vi "Increment Filename changename.vi"(8 "error in (no error)":errorcluster, 11 "path":path=path "C:/user/patrick/test/test/filename.itx") -> (0 "error out":errorcluster, 3 "modified path":path=path "C:/")   [LabVIEW 2016]
panel:
  out "Numeric":i32
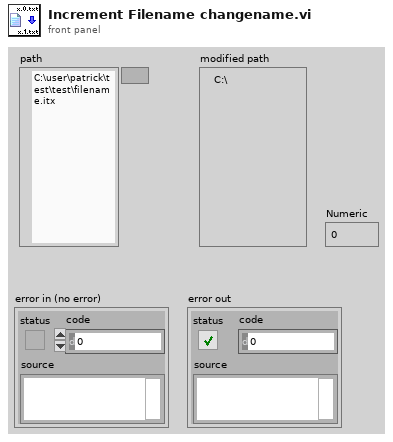
[diagram p1: front panel]
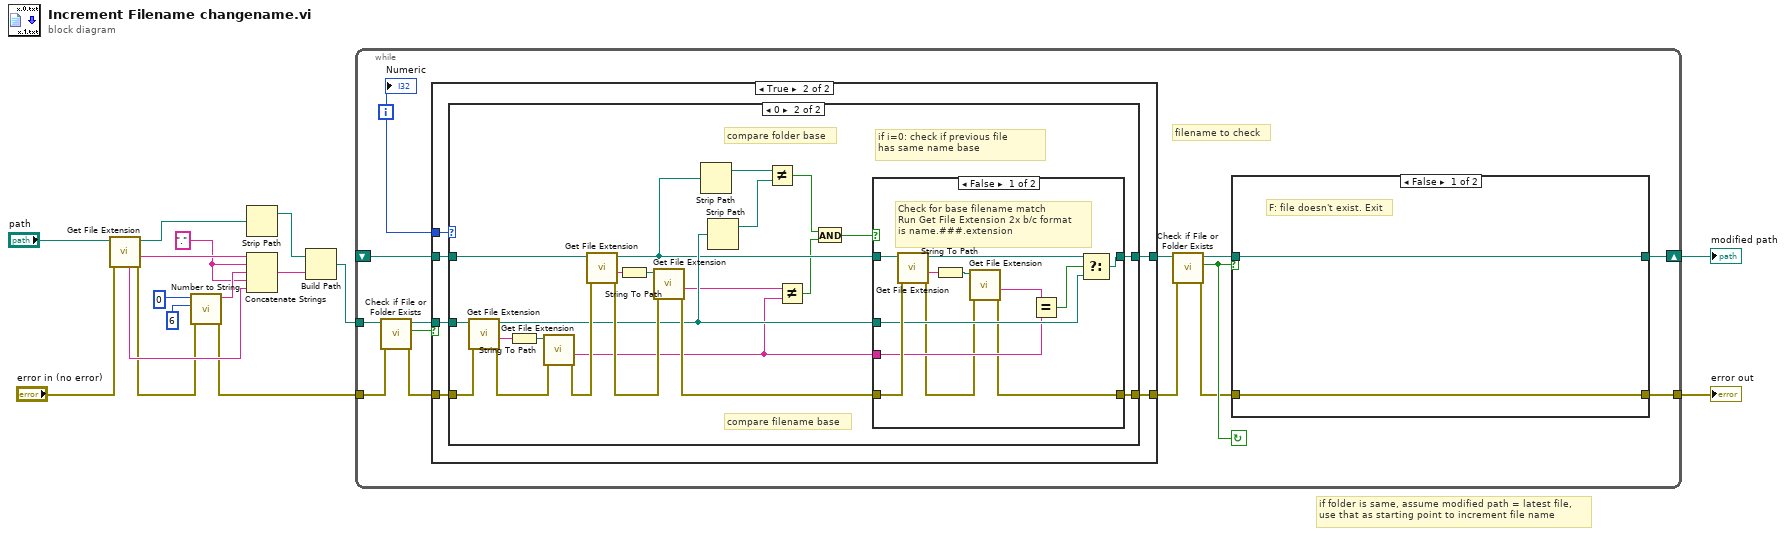
[diagram p0: block diagram]
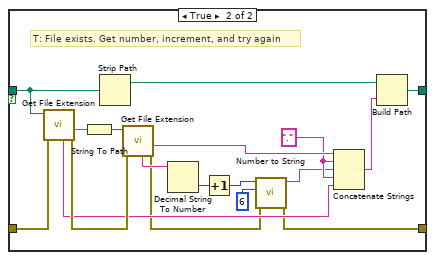
[diagram p5: hidden frame]
diagram:
  w4 = "."
  # "if folder is same, assume modified path = latest file,\nuse that as starting point to increment file name"
  n1 = call <vilib>:"Get File Extension.vi"("error in (no error)"="error in (no error)", "file"="path") -> ("error out"=w3:errorcluster, "filename without extension"=w11:string, "dup file"=w15:path, "unmodified file extension"=w8:string)  [unwired: 6 out]
  n2 = call "Number to String.vi"("error in (no error)"=w3, "desired minimum string length"=6, "number"=0) -> ("error out"=w2:errorcluster, "String"=w5:string)  [unwired: 7 in]
  n3 = Strip Path(path=w15) -> (stripped path=w7:path)  [unwired: 1 out]
  n4 = Concatenate Strings(w11, w4, w5, w4, w8) -> (w14:string)
  n5 = Build Path(base path=w7, name or relative path=w14) -> (appended path=w9:path)
  n6 = while {
    shift-right: [w28] -> w13
    shift-left: _ -> [w23]
    tunnel: w2 -> [w19]
    tunnel: [w26] -> w10
    tunnel: w9 -> [w20]
    i -> [w22]
    stop <- w29 continue-if-true
    # "filename to check"
    n7 = call <vilib>:"Check if File or Folder Exists.vi"("error in (no error)"=w19, "path"=w20) -> ("error out"=w18:errorcluster, "file or folder exists?"=w17:bool, "dup path"=w21:path)  [unwired: 7 out]
    n8 = case shown="True" w17 {
      tunnel: [w32 w38] -> w25
      tunnel: [w31 w37] -> w24
      tunnel: w23 -> [_ w36]
      tunnel: w22 -> [_ w35]
      tunnel: w21 -> [w31 w34]
      tunnel: w18 -> [w32 w33]
      frame False {
        # "If file.000000.* doesn't exist, just skip this step"
      }
      frame True {
        n9 = case shown="0" w35 {
          tunnel: [w39 w62] -> w38
          tunnel: w34 -> [_ w56]
          tunnel: w33 -> [w39 w61]
          tunnel: [w40 w60] -> w37
          tunnel: w36 -> [w40 w53]
          frame Default {
            # "if i>0, you can't use previous file and you're going to have to scan through\nthe entire directory"
          }
          frame 0 {
            # "compare filename base"
            # "compare folder base"
            # "if i=0: check if previous file\nhas same name base"
            n10 = call <vilib>:"Get File Extension.vi"("error in (no error)"=w61, "file"=w56) -> ("error out"=w57:errorcluster, "filename without extension"=w58:string, "dup file"=w47:path)  [unwired: 7 out]
            n11 = String To Path(string=w58) -> (path=w59:path)
            n12 = call <vilib>:"Get File Extension.vi"("error in (no error)"=w57, "file"=w59) -> ("error out"=w50:errorcluster, "filename without extension"=w44:string)  [unwired: 8 out]
            n13 = call <vilib>:"Get File Extension.vi"("error in (no error)"=w50, "file"=w53) -> ("error out"=w48:errorcluster, "filename without extension"=w52:string, "dup file"=w46:path)  [unwired: 7 out]
            n14 = String To Path(string=w52) -> (path=w51:path)
            n15 = call <vilib>:"Get File Extension.vi"("error in (no error)"=w48, "file"=w51) -> ("error out"=w49:errorcluster, "filename without extension"=w45:string)  [unwired: 8 out]
            n16 = Strip Path(path=w46) -> (stripped path=w54:path)  [unwired: 1 out]
            n17 = Strip Path(path=w47) -> (stripped path=w55:path)  [unwired: 1 out]
            n18 = Not Equal?(x=w54, y=w55) -> (x != y?=w41:bool)
            n19 = Not Equal?(x=w45, y=w44) -> (x != y?=w43:bool)
            n20 = And(x=w41, y=w43) -> (x .and. y?=w42:bool)
            n21 = case shown="False" w42 {
              tunnel: [w64 w75] -> w62
              tunnel: w44 -> [w68 _]
              tunnel: w49 -> [w74 w75]
              tunnel: w47 -> [w71 w76]
              tunnel: w46 -> [w70 _]
              tunnel: [w69 w76] -> w60
              frame False {
                # "Check for base filename match\nRun Get File Extension 2x b/c format\nis name.###.extension"
                n22 = call <vilib>:"Get File Extension.vi"("error in (no error)"=w74, "file"=w70) -> ("error out"=w65:errorcluster, "filename without extension"=w66:string, "dup file"=w73:path)  [unwired: 7 out]
                n23 = String To Path(string=w66) -> (path=w67:path)
                n24 = call <vilib>:"Get File Extension.vi"("error in (no error)"=w65, "file"=w67) -> ("error out"=w64:errorcluster, "filename without extension"=w63:string)  [unwired: 8 out]
                n25 = Equal?(x=w63, y=w68) -> (x = y?=w72:bool)
                n26 = Select(t=w73, s=w72, f=w71) -> (s? t:f=w69:path)
              }
              frame True {
                # "If no previous file use new one"
              }
            }
          }
        }
      }
    }
    n27 = call <vilib>:"Check if File or Folder Exists.vi"("error in (no error)"=w25, "path"=w24) -> ("error out"=w27:errorcluster, "file or folder exists?"=w29:bool, "dup path"=w30:path)  [unwired: 7 out]
    n28 = case shown="False" w29 {
      tunnel: w30 -> [w78 w96]
      tunnel: [w78 w95] -> w28
      tunnel: w27 -> [w77 w87]
      tunnel: [w77 w80] -> w26
      frame False {
        # "F: file doesn't exist. Exit"
      }
      frame True {
        w91 = "." ("regular expression")
        # "T: File exists. Get number, increment, and try again"
        n29 = call <vilib>:"Get File Extension.vi"("error in (no error)"=w87, "file"=w96) -> ("error out"=w86:errorcluster, "filename without extension"=w85:string, "unmodified file extension"=w84:string)  [unwired: 7 out]
        n30 = String To Path(string=w85) -> (path=w93:path)
        n31 = Strip Path(path=w96) -> (stripped path=w88:path)  [unwired: 1 out]
        n32 = call <vilib>:"Get File Extension.vi"("error in (no error)"=w86, "file"=w93) -> ("error out"=w81:errorcluster, "filename without extension"=w92:string, "unmodified file extension"=w83:string)  [unwired: 7 out]
        n33 = Decimal String To Number(string=w83) -> (number=w89:i32)  [unwired: 1 in, 2 out]
        n34 = Increment(x=w89) -> (x+1=w90:i32)
        n35 = call "Number to String.vi"("error in (no error)"=w81, "desired minimum string length"=6, "number"=w90) -> ("error out"=w80:errorcluster, "String"=w82:string)  [unwired: 7 in]
        n36 = Concatenate Strings(w92, w91, w82, w91, w84) -> (w94:string)
        n37 = Build Path(base path=w88, name or relative path=w94) -> (appended path=w95:path)
      }
    }
    "Numeric" <- w22
  }
  "modified path" <- w13
  "error out" <- w10
